vi "Heater Sensor.vi"() -> ()   [LabVIEW 2021]
uses:
  <vilib>/MakerHub/LINX/Public/Peripherals/Analog/Analog Read 1 Chan.vi
  <vilib>/MakerHub/LINX/Public/Peripherals/Digital/Digital Write 1 Chan.vi
  <vilib>/MakerHub/LINX/Public/Peripherals/Analog/Analog Read N Chans.vi
  <vilib>/MakerHub/LINX/Public/Peripherals/Digital/Digital Write N Chans.vi
  <vilib>/MakerHub/LINX/Private/Local IO/LinxAnalogRead.vi
  <vilib>/MakerHub/LINX/Public/Utilities/Check Channel.vi
  <vilib>/MakerHub/LINX/Private/Local IO/LinxDigitalWrite.vi
  <vilib>/MakerHub/LINX/Public/Utilities/Open Serial.vi
  <vilib>/MakerHub/LINX/Private/Utilties/Generate Error.vi
  <vilib>/MakerHub/LINX/LMH-LINX.lvlib
panel:
  out "Heater On":bool
  out "Temperature":dbl
  out "Thermometer":dbl(slide) scale=0.0..100.0
  in  "Thermistor resistance at room temp":dbl
  in  "Thermistor Room Temp":dbl
  in  "B rating":dbl
  in  "Resistor":dbl
  in  "Target Temp":dbl
  in  "Analog Channel":u8
  in  "DO Channel":u8
  in  "Serial Port":refnum<visa-resource-name>="N/A"
  in  "Stop":bool
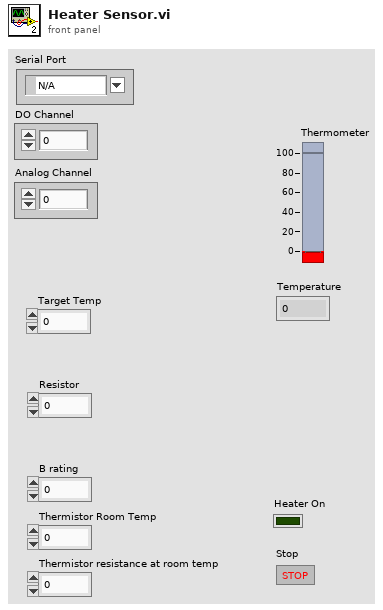
[diagram p1: front panel]
types:
  T1 = typedef "LMH-LINX.lvlib/LINX Ref.ctl" = cluster{"IO":T2, "Interface":T3, "LINX Device Config":T4}
  T2 = typedef "LMH-LINX.lvlib/Platform.ctl" = enum16{"Remote", "Local"}
  T3 = typedef "LMH-LINX.lvlib/Interface.ctl" = enum16{"Serial", "TCP"}
  T4 = typedef "LMH-LINX.lvlib/Device.lvlib/LINX Device Config.ctl" = cluster{"Interface":T3, "COM Port":refnum<visa-resource-name>, "TCP Configuration":T5, "Device Family":u8, "Device ID":u8, "Device Name":string, "TCP Ref":refnum<k5>, "Channels":T6}
  T5 = typedef "LMH-LINX.lvlib/Device.lvlib/TCP Config.ctl" = cluster{"IP Address":string, "Port":u16}
  T6 = typedef "LMH-LINX.lvlib/Channels.ctl" = cluster{"DI":u8[], "DO":u8[], "AI":u8[], "AO":u8[], "PWM":u8[], "QE":u8[], "UART":u8[], "I2C 2":u8[], "SPI":u8[], "CAN":u8[], "Servo":u8[], "AI Ref (V)":dbl, "AI Resolution (Bits)":u8, "AO Ref (V)":dbl, "AO Resolution (Bits)":u8}
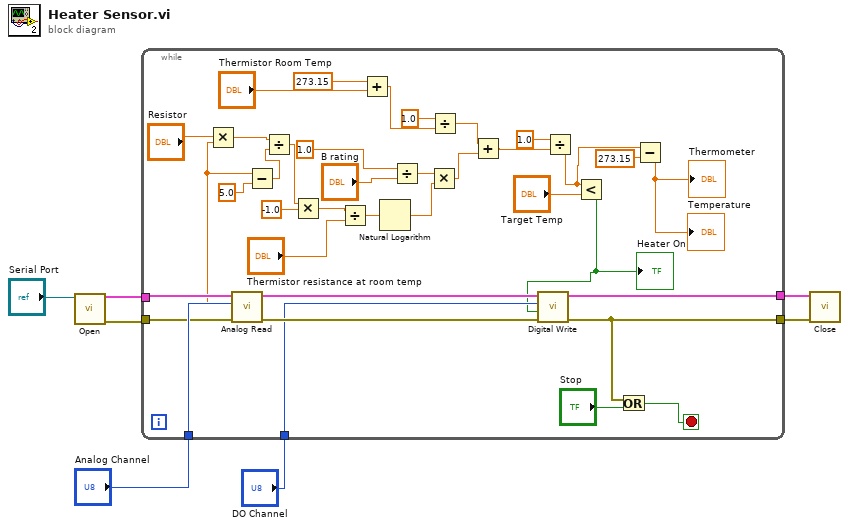
[diagram p0: block diagram]
diagram:
  n1 = call-poly <vilib>:"Open.vi"("Serial Port"="Serial Port") -> ("Error Out"=w5:errorcluster, "LINX Resource"=w7:T1)  [unwired: 8 in, 1 out]
  n2 = while {
    tunnel: w7 -> [w35]
    tunnel: [w44] -> w6
    tunnel: w5 -> [w37]
    tunnel: [w42] -> w4
    tunnel: "Analog Channel" -> [w40]
    tunnel: "DO Channel" -> [w36]
    stop <- w41 stop-if-true
    n3 = call-poly <vilib>:"Analog Read.vi"("Error In"=w37, "Analog Channel"=w40, "LINX Resource"=w35) -> ("Error Out"=w38:errorcluster, "Voltage"=w32:dbl, "LINX Resource"=w39:T1)  [unwired: 5 in, 1 out]
    n4 = Multiply(x="Resistor", y=w32) -> (x*y=w34:dbl)
    n5 = Subtract(x=w32, y=5.0) -> (x-y=w33:dbl)
    n6 = Divide(x=w34, y=w33) -> (x/y=w12:dbl)
    n7 = Multiply(x=w12, y=-1.0) -> (x*y=w14:dbl)
    n8 = Divide(x=w14, y="Thermistor resistance at room temp") -> (x/y=w29:dbl)
    n9 = Add(x=273.15, y="Thermistor Room Temp") -> (x+y=w19:dbl)
    n10 = Natural Logarithm(1:w29) -> (0:w30:dbl)
    n11 = Divide(x=1.0, y="B rating") -> (x/y=w22:dbl)
    n12 = Multiply(x=w22, y=w30) -> (x*y=w28:dbl)
    n13 = Divide(x=1.0, y=w19) -> (x/y=w18:dbl)
    n14 = Add(x=w18, y=w28) -> (x+y=w27:dbl)
    n15 = Divide(x=1.0, y=w27) -> (x/y=w10:dbl)
    n16 = Less?(x=w10, y="Target Temp") -> (x < y?=w8:bool)
    "Heater On" <- w8
    n17 = call-poly <vilib>:"Digital Write.vi"("Error In"=w38, "Output Value"=w8, "DO Channel"=w36, "LINX Resource"=w39) -> ("Error Out"=w42:errorcluster, "LINX Resource"=w44:T1)  [unwired: 6 in]
    n18 = Or(x=w42, y="Stop") -> (x .or. y?=w41:bool)
    n19 = Subtract(x=w10, y=273.15) -> (x-y=→"Thermometer" →"Temperature":dbl)
  }
  n20 = call <vilib>:"Close.vi"("Error In"=w4, "LINX Resource"=w6) -> ()  [unwired: 9 in, 1 out]
